vi "WorkingSimplexonDummyData.vi"() -> ()   [LabVIEW 2019]
uses:
  <vilib>/gmath/NumericalOptimization/stopping criteria.ctl
  <vilib>/gmath/NumericalOptimization/Downhill Simplex.vi
  <vilib>/gmath/NI_Gmath.lvlib
panel:
  in  "Combo Box":string(combo)
  out "x-y":dbl
  in  "stopping criteria":T1={"function tolerance"=1e-06, "parameter tolerance"=1e-06, "max iterations"=100, "max function calls"=1000, "gradient tolerance"=1e-06, "max time (sec)"=-1.0}
  out "number of function evaluations":i32
  out "f(minimum)":dbl
  out "minimum":dbl[](array[numeric])
  out "XY Intensity Map":dbl[][](graph)
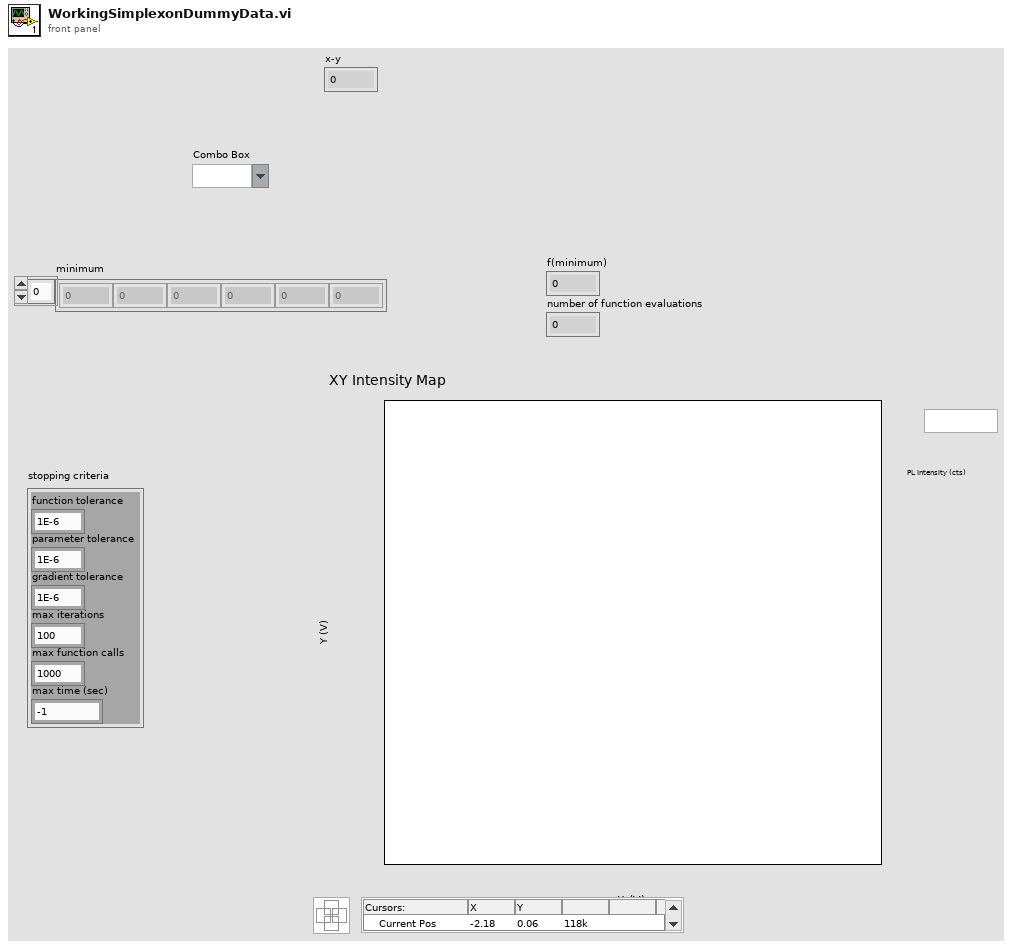
[diagram p1: front panel]
types:
  T1 = typedef "NI_Gmath.lvlib/stopping criteria.ctl" = cluster{"function tolerance":dbl, "parameter tolerance":dbl, "max iterations":i32, "max function calls":i32, "gradient tolerance":dbl, "max time (sec)":dbl}
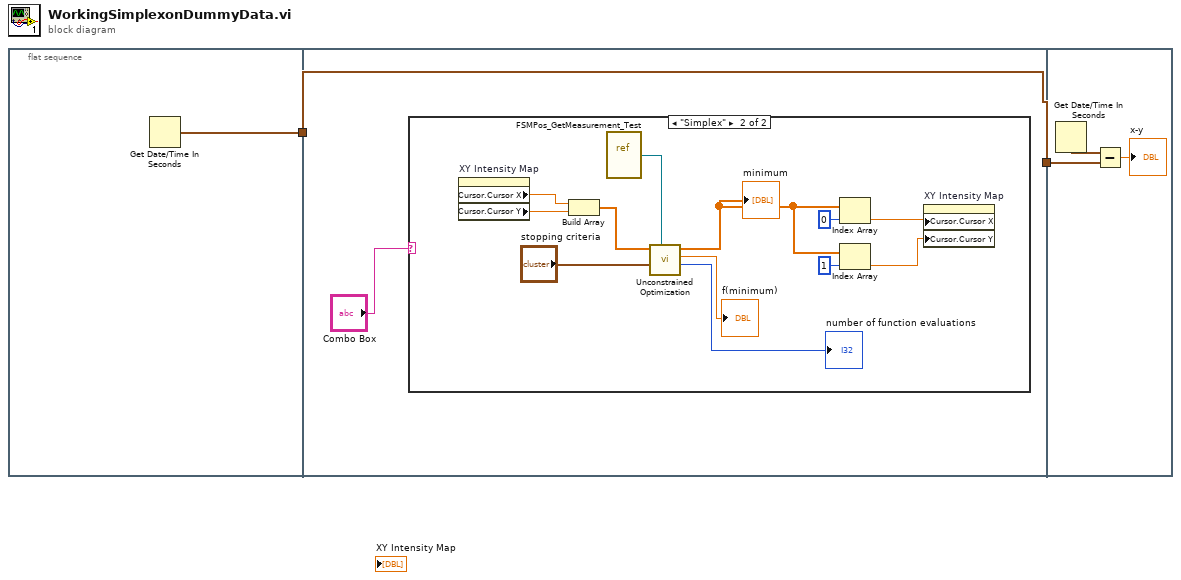
[diagram p0: block diagram]
diagram:
  n1 = flat-sequence {
    tunnel: [w3] -> w2
    tunnel: w2 -> [w5]
    tunnel: [w5] -> w1
    tunnel: w1 -> [w19]
    frame #0 {
      n2 = Get Date/Time In Seconds() -> (seconds since 1Jan1904=w3:timestamp)
    }
    frame #1 {
      n3 = case shown="\"Simplex\"" "Combo Box" {
        frame "Hill method", Default {
        }
        frame "Simplex" {
          n4 = property on="XY Intensity Map" class="IntGraph (strict)"() -> ("Cursor.Cursor X"=w17:dbl, "Cursor.Cursor Y"=w16:dbl)  [unwired: 2 in, 2 out]
          n5 = Build Array(w17, w16) -> (w7:dbl[])
          n6 = vi-ref "FSMPos_GetMeasurement_Test.vi"() -> (w6:refnum<vi>)
          n7 = call-poly <vilib>:"Unconstrained Optimization.vi"("objective function"=w6, "stopping criteria"="stopping criteria", "start"=w7) -> ("number of function evaluations"=→"number of function evaluations":i32, "f(minimum)"=→"f(minimum)":dbl, "minimum"=w10:dbl[])  [unwired: 5 in, 1 out]
          "minimum" <- w10
          n8 = Index Array(array=w10, index=0) -> (element=w12:dbl)
          n9 = Index Array(array=w10, index=1) -> (element=w9:dbl)
          n10 = property on="XY Intensity Map" class="IntGraph (strict)"("Cursor.Cursor X"=w12, "Cursor.Cursor Y"=w9) -> ()  [unwired: 2 in, 2 out]
        }
      }
    }
    frame #2 {
      n11 = Get Date/Time In Seconds() -> (seconds since 1Jan1904=w20:timestamp)
      n12 = Subtract(x=w20, y=w19) -> (x-y=→"x-y":dbl)
    }
  }
